vi "relative move from offset and calibration.vi"(6 "Cal neg":dbl, 9 "Cal":dbl, 10 "Offset":dbl, 11 "Invert Direction":bool) -> (3 "relative move out":dbl)   [LabVIEW 2020]
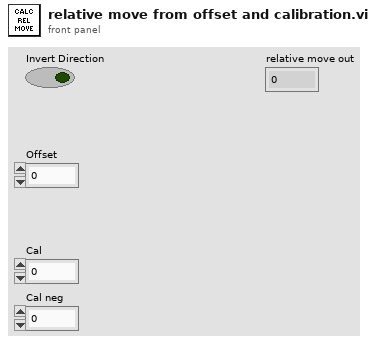
[diagram p1: front panel]
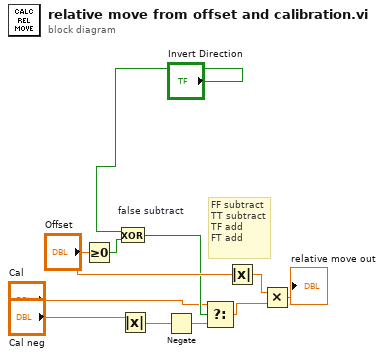
[diagram p0: block diagram]
diagram:
  # "FF subtract\nTT subtract\nTF add\nFT add"
  n1 = Greater Or Equal To 0?(x="Offset") -> (x >= 0?=w5:bool)
  n2 = Exclusive Or "false subtract"(1:w5, 2:"Invert Direction") -> (0:w6:bool)
  n3 = Absolute Value(x="Cal neg") -> (abs(x)=w11:dbl)
  n4 = Negate(x=w11) -> (-x=w9:dbl)
  n5 = Select(t="Cal", s=w6, f=w9) -> (s? t:f=w3:dbl)
  n6 = Absolute Value(x="Offset") -> (abs(x)=w8:dbl)
  n7 = Multiply(x=w8, y=w3) -> (x*y=→"relative move out":dbl)
